vi "Exclude Test Methods from Code Coverage.vi"(11 "Code Coverage":map{path, dbl}(c390)) -> (3 "Filtered Code Coverage":map{path, dbl}(c390))   [LabVIEW 2020, in "LUnit Tests.lvlib" / "Coverage Test.lvclass"]
uses:
  Coverage Test.lvclass
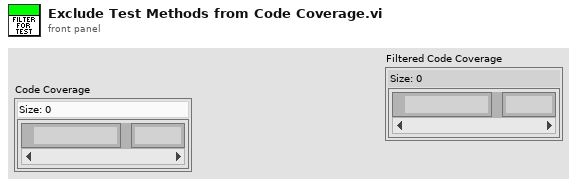
[diagram p1: front panel]
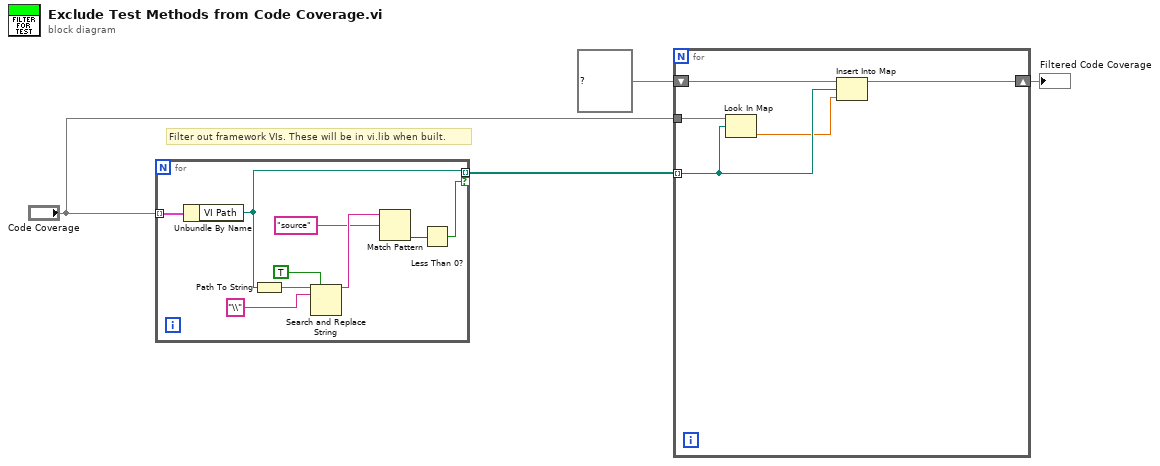
[diagram p0: block diagram]
diagram:
  # "Filter out framework VIs. These will be in vi.lib when built."
  n1 = for {
    tunnel: "Code Coverage" -> [w13] mode=indexing
    tunnel: [w11] -> w1 mode=indexing if=w9
    n2 = Unbundle By Name(w13) -> ("VI Path"=w11:path)
    n3 = Path To String(path=w11) -> (string=w12:string)
    n4 = Search and Replace String(replace all?=TRUE ("replace all? (F)"), input string=w12, search string="\\") -> (result string=w8:string)  [unwired: 5 in, 3 out]
    n5 = Match Pattern(string=w8, regular expression="source") -> (offset past match=w10:i32)  [unwired: 1 in, 3 out]
    n6 = Less Than 0?(x=w10) -> (x < 0?=w9:bool)
  }
  n7 = for {
    shift-right: [w17] -> w2
    shift-left: map{path, dbl} {} ("Code Coverage") -> [w18]
    tunnel: w1 -> [w15] mode=indexing
    tunnel: "Code Coverage" -> [w16]
    n8 = Look In Map(map=w16, key=w15) -> (value=w14:dbl)  [unwired: 1 in, 1 out]
    n9 = Insert Into Map(map in=w18, key=w15, value=w14) -> (map out=w17:map{path, dbl})  [unwired: 2 out]
  }
  "Filtered Code Coverage" <- w2
